vi "APS write d channel output.vi"(0 "Board_ID":i32, 2 "DO_Group":i32, 4 "字符串":string, 5 "error in (no error)":errorcluster caption="错误输入（无错误）", 8 "布尔":bool=TRUE) -> (14 "function return":i32, 19 "error out":errorcluster caption="错误输出")   [LabVIEW 2014, in "APS168.lvlib"]
doc: "I32 FNTYPE APS_write_d_channel_output(I32 Board_ID, I32 DO_Group, I32 Ch_No, I32 DO_Data);"
uses:
  APS168.lvlib
  APS168.dll
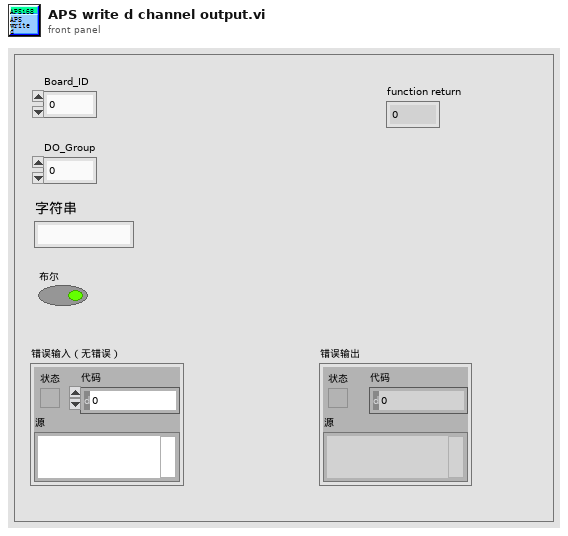
[diagram p1: front panel]
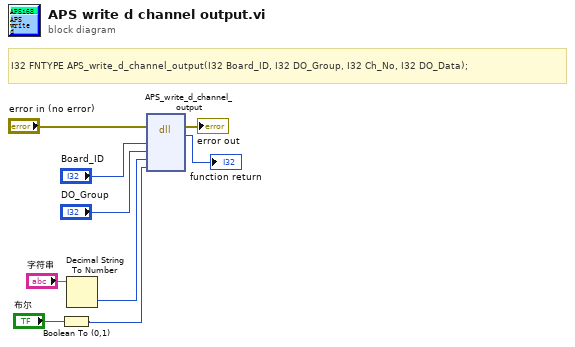
[diagram p0: block diagram]
diagram:
  # "I32 FNTYPE APS_write_d_channel_output(I32 Board_ID, I32 DO_Group, I32 Ch_No, I32 DO_Data);"
  n1 = Boolean To (0,1)(Boolean="布尔") -> (0, 1=w3:i16)
  n2 = Decimal String To Number(string="字符串") -> (number=w1:i32)  [unwired: 2 in, 1 out]
  n3 = dll-call lib="PTH2Eabs F称重称重SubviADLINKLLB运动204c\nAPS168.dll" fn="APS_write_d_channel_output"(error in="error in (no error)", "Board_ID"="Board_ID", "DO_Group"="DO_Group", "Ch_No"=w1, "DO_Data"=w3) -> (error out=→"error out":errorcluster, "返回类型"=→"function return":i32)  [unwired: 6 in, 1 out]
